vi "(SubVI) Difference calculater_YCC.vi"(3 "T= (i+1)-i\nF=i-(i+1)":bool, 4 "Array in":dbl[](array[numeric])) -> (1 "Diff":dbl[](array[numeric]))   [LabVIEW 2014]
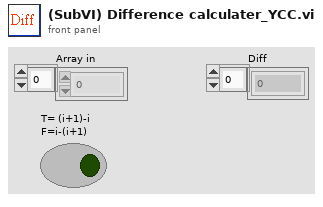
[diagram p1: front panel]
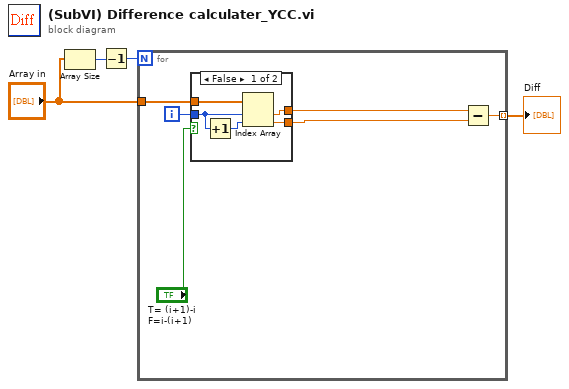
[diagram p0: block diagram]
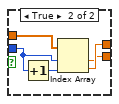
[diagram p2: hidden frame]
diagram:
  n1 = Array Size(array="Array in") -> (size(s)=w2:i32)
  n2 = Decrement(x=w2) -> (x-1=w3:i32)
  n3 = for {
    N: w3 -> [_]
    tunnel: "Array in" -> [w6]
    tunnel: [w9] -> w4 mode=indexing
    i -> [w10]
    n4 = case shown="False" "T= (i+1)-i\nF=i-(i+1)" {
      tunnel: w10 -> [w14 w19]
      tunnel: [w13 w17] -> w8
      tunnel: [w12 w16] -> w7
      tunnel: w6 -> [w11 w18]
      frame False {
        n5 = Increment(x=w14) -> (x+1=w15:i32)
        n6 = Index Array(array=w11, index #1=w14, index #2=w15) -> (element #1=w13:dbl, element #2=w12:dbl)
      }
      frame True {
        n7 = Increment(x=w19) -> (x+1=w20:i32)
        n8 = Index Array(array=w18, index #1=w19, index #2=w20) -> (element #1=w16:dbl, element #2=w17:dbl)
      }
    }
    n9 = Subtract(x=w8, y=w7) -> (x-y=w9:dbl)
  }
  "Diff" <- w4
